vi "Calculate Adjacent Points.vi"(5 "End Point":cluster{"X":dbl, "Y":dbl}={"X"=10.0, "Y"=5.0}, 6 "Closed List In":T1(array[cluster]), 7 "Blocked Points":cluster{"X":dbl, "Y":dbl}[](array[cluster]), 8 "error in (no error)":errorcluster, 10 "Open Point":cluster{"X":dbl, "Y":dbl}={"X"=0.0, "Y"=5.0}, 11 "Open List In":T1(array[cluster])) -> (0 "error out":errorcluster, 2 "Open List Out":T1(array[cluster]), 4 "End Point Out":cluster{"X":dbl, "Y":dbl}={"X"=10.0, "Y"=5.0})   [LabVIEW 2009]
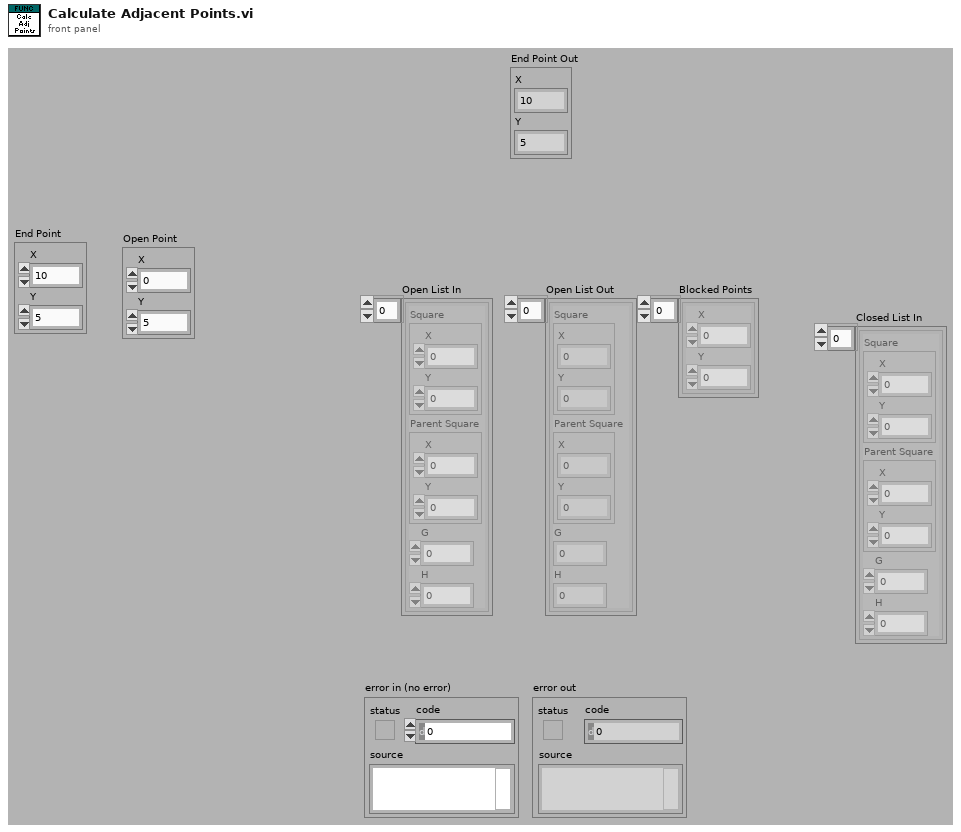
[diagram p1: front panel]
types:
  T1 = cluster{"Square":cluster{"X":dbl, "Y":dbl}, "Parent Square":cluster{"X":dbl, "Y":dbl}, "G":dbl, "H":dbl}[]
  T2 = cluster{"Square":cluster{"X":dbl, "Y":dbl}, "Parent Square":cluster{"X":dbl, "Y":dbl}, "G":dbl, "H":dbl}
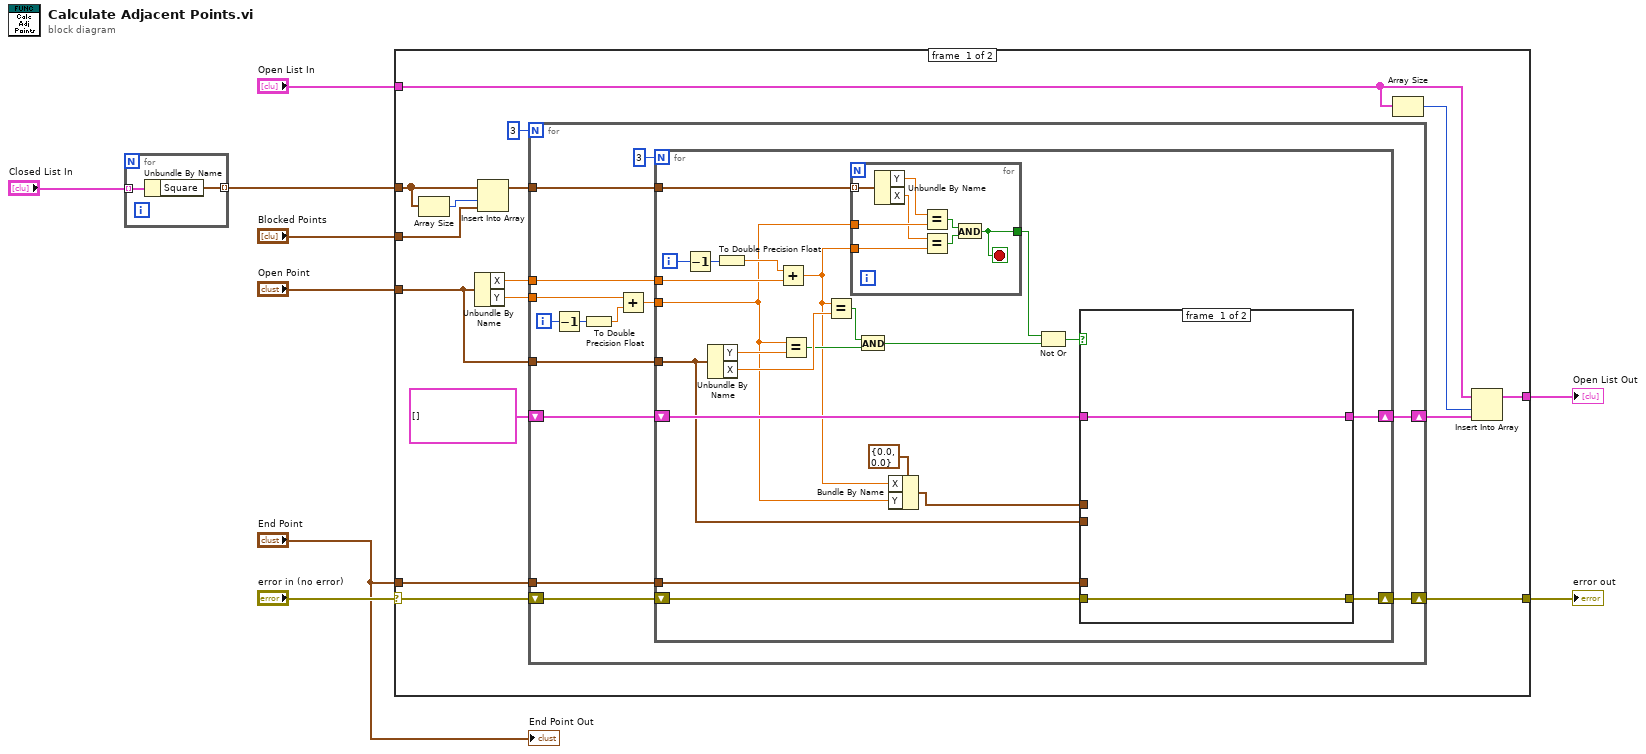
[diagram p0: block diagram]
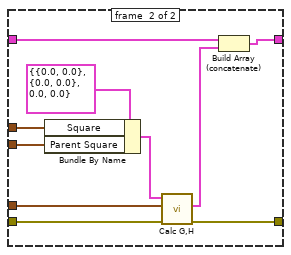
[diagram p2: hidden frame]
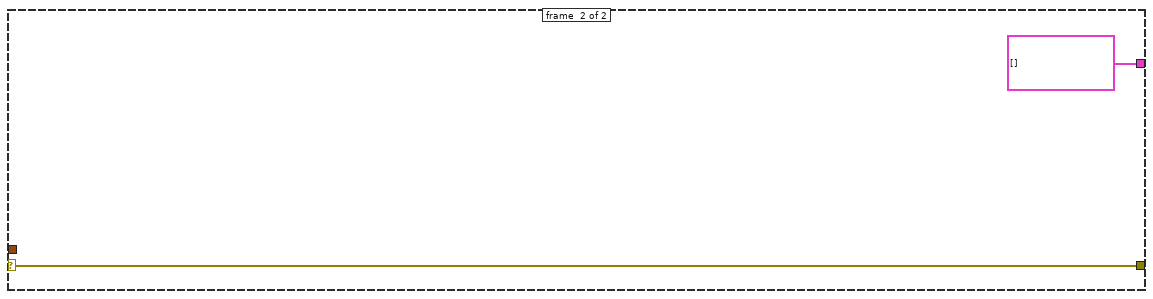
[diagram p3: hidden frame]
diagram:
  n1 = for {
    tunnel: "Closed List In" -> [w11] mode=indexing
    tunnel: [w10] -> w1 mode=indexing
    n2 = Unbundle By Name(w11) -> ("Square"=w10:cluster{"X":dbl, "Y":dbl})
  }
  n3 = case shown="No Error" "error in (no error)" {
    selector: "error in (no error)" -> [w22 w85]
    tunnel: "Open Point" -> [w25 _]
    tunnel: "End Point" -> [w21 _]
    tunnel: [w20 w85] -> w6
    tunnel: "Open List In" -> [w19 _]
    tunnel: [w16 T1 [] ("Open List In")] -> w4
    tunnel: "Blocked Points" -> [w13 _]
    tunnel: w1 -> [w15 _]
    frame #0 {
      n4 = Array Size(array=w15) -> (size(s)=w14:i32)
      n5 = Unbundle By Name(w25) -> ("X"=w27:dbl, "Y"=w26:dbl)
      n6 = Insert Into Array(array=w15, index=w14, new element=w13) -> (w12:cluster{"X":dbl, "Y":dbl}[])
      n7 = for {
        N: 3 -> [_]
        tunnel: w27 -> [w38]
        tunnel: w26 -> [w41]
        tunnel: w25 -> [w37]
        shift-right: [w35] -> w17
        shift-left: T1 [] -> [w36]
        tunnel: w21 -> [w30]
        shift-right: [w29] -> w20
        shift-left: w22 -> [w31]
        tunnel: w12 -> [w28]
        i -> [w34]
        n8 = Decrement(x=w34) -> (x-1=w33:i32)
        n9 = To Double Precision Float(number=w33) -> (double precision float=w40:dbl)
        n10 = Add(x=w41, y=w40) -> (x+y=w39:dbl)
        n11 = for {
          N: 3 -> [_]
          tunnel: w39 -> [w46]
          tunnel: w38 -> [w62]
          tunnel: w37 -> [w55]
          shift-right: [w53] -> w35
          shift-left: w36 -> [w57]
          tunnel: w30 -> [w48]
          shift-right: [w50] -> w29
          shift-left: w31 -> [w49]
          tunnel: w28 -> [w47]
          i -> [w52]
          n12 = Decrement(x=w52) -> (x-1=w51:i32)
          n13 = Unbundle By Name(w55) -> ("Y"=w60:dbl, "X"=w61:dbl)
          n14 = To Double Precision Float(number=w51) -> (double precision float=w63:dbl)
          n15 = Add(x=w63, y=w62) -> (x+y=w45:dbl)
          n16 = Equal?(x=w46, y=w60) -> (x = y?=w59:bool)
          n17 = Equal?(x=w45, y=w61) -> (x = y?=w58:bool)
          n18 = for {
            tunnel: w47 -> [w71] mode=indexing
            tunnel: w46 -> [w69]
            tunnel: w45 -> [w67]
            tunnel: [w64] -> w43
            stop <- w64 stop-if-true
            n19 = Unbundle By Name(w71) -> ("Y"=w70:dbl, "X"=w68:dbl)
            n20 = Equal?(x=w70, y=w69) -> (x = y?=w66:bool)
            n21 = Equal?(x=w68, y=w67) -> (x = y?=w65:bool)
            n22 = And(x=w66, y=w65) -> (x .and. y?=w64:bool)
          }
          n23 = And(x=w58, y=w59) -> (x .and. y?=w44:bool)
          n24 = Bundle By Name(cluster=cluster{"X":dbl, "Y":dbl} {"X"=0.0, "Y"=0.0} ("Square"), "X"=w45, "Y"=w46) -> (w54:cluster{"X":dbl, "Y":dbl})
          n25 = Not Or(1:w44, 2:w43) -> (0:w42:bool)
          n26 = case shown="True" w42 {
            tunnel: w57 -> [w73 w83]
            tunnel: w54 -> [_ w82]
            tunnel: w55 -> [_ w81]
            tunnel: [w73 w80] -> w53
            tunnel: [w72 w76] -> w50
            tunnel: w49 -> [w72 w78]
            tunnel: w48 -> [_ w77]
            frame #0 {
            }
            frame #1 {
              n27 = Bundle By Name(cluster=T2 {"Square"={"X"=0.0, "Y"=0.0}, "Parent Square"={"X"=0.0, "Y"=0.0}, "G"=0.0, "H"=0.0} ("Cluster"), "Square"=w82, "Parent Square"=w81) -> (w75:T2)
              n28 = call "Calc G,H.vi"("error in (no error)"=w78, "End Point"=w77, "Square In"=w75) -> ("error out"=w76:errorcluster, "Square Out"=w74:T2)  [unwired: 7 in]
              n29 = Build Array (concatenate)(w83, w74) -> (w80:T1)
            }
          }
        }
      }
      n30 = Array Size(array=w19) -> (size(s)=w18:i32)
      n31 = Insert Into Array(array=w19, index=w18, new element=w17) -> (w16:T1)
    }
    frame #1 {
    }
  }
  "error out" <- w6
  "Open List Out" <- w4
  "End Point Out" <- "End Point"
